vi "Disconnect.vi"(8 "error in (no error)":errorcluster, 11 "HRS_Spectrometer in":refnum<class "HRS_Spectrometer.lvclass">) -> (0 "error out":errorcluster, 3 "HRS_Spectrometer out":refnum<class "HRS_Spectrometer.lvclass">)   [LabVIEW 2023, in "HRS_Spectrometer.lvlib" / "HRS_Spectrometer.lvclass"]
uses:
  HRS_Spectrometer.lvclass
  HRS_Spectrometer.lvclass/HRS_Spectrometer.ctl
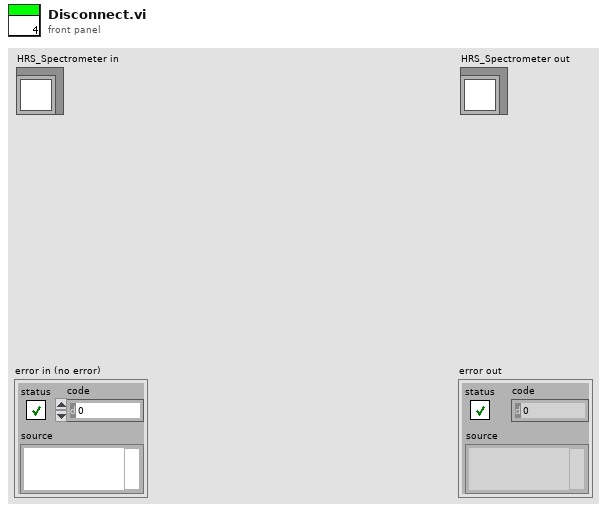
[diagram p1: front panel]
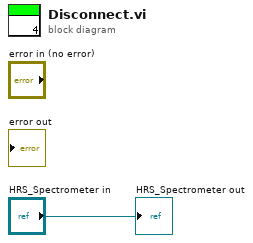
[diagram p0: block diagram]
diagram:
  "HRS_Spectrometer out" <- "HRS_Spectrometer in"
